vi "Write Data to HW.vi"(11 "Plugin in":refnum<class "Plugin.lvclass">) -> (0 "error out":errorcluster, 3 "Plugin out":refnum<class "Plugin.lvclass">)   [LabVIEW 2024, in "FPGA Addon Engine.lvlib" / "Plugin.lvclass"]
uses:
  Plugin.lvclass
  Plugin.lvclass/Plugin.ctl
  FPGA Addon Engine.lvlib
  VS Engine Abstraction/VS Engine Interface/VS Engine Interface.lvclass
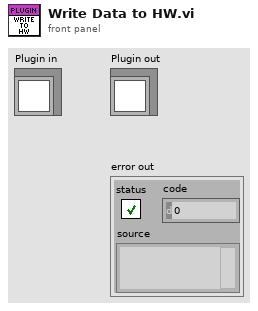
[diagram p1: front panel]
types:
  T1 = typedef "FPGA Addon Engine.lvlib/State Variables.ctl" = cluster{"FPGA Ref":refnum<k20>, "IncomingRegisters.Refs":T2[], "IncomingDMA.Refs":T5[], "OutgoingRegisters.Refs":T2[], "OutgoingDMA.Refs":T10[], "Compiled":T12}
  T2 = typedef "FPGA Addon Engine.lvlib/Register Settings.ctl" = cluster{"Name":string, "Data Type":T3, "session":u32, "Scalar Type":T4, "Index":i32, "Length":i32, "attributes":variant, "default value":variant, "RegisterOffset":u32}
  T3 = typedef "FPGA Addon Shared.lvlib/FPGA Addon Data Type.ctl" = enum8{"<Null>", "I8", "I16", "I32", "I64", "U8", "U16", "U32", "U64", "SGL", "Boolean", "Analog PWM In Settings", "Analog PWM In", "Digital PWM In Settings", "Digital PWM In", "Digital PWM Out", "Sine Out", "FXP", "FXP+/-24.5", "FXP+/-16.5", "FXP+/-32.8", "FXP+/-64.32", "FXP+/-16.7", "FXP+/-20.5", "FXP+/-27.5", "FXP+/-32.16", "FXP+16.3", "FXP+18.3", "Digital Static In", "Digital Static Out", "Digital Static In Settings", "Digital WSS Out", "Quad Encoder Settings", "Quad Encoder In", "Group"}
  T4 = typedef "FPGA Addon Shared.lvlib/Scalar Type.ctl" = enum16{"Standard", "Bitpacked"}
  T5 = typedef "FPGA Addon Engine.lvlib/DMA Input References.ctl" = cluster{"Addon Name":string, "Waveform Ref":refnum<class "Multiple Waveforms Write (DBL).lvclass">, "DMA Name":string, "DMA Settings":T6, "Refs":T9}
  T6 = typedef "FPGA Addon Shared.lvlib/DMA Settings.ctl" = cluster{"Number of Channels":u8, "Delacing Scheme":T7, "Update Rate":u32, "dt":dbl, "Mode":T8, "Number of Samples":u32, "DMA Host Buffer":u32}
  T7 = typedef "FPGA Addon Shared.lvlib/Delacing Scheme.ctl" = enum8{"Interleaved", "Bitpacked"}
  T8 = typedef "FPGA Addon Shared.lvlib/DMA Acquisition Mode.ctl" = enum8{"Continuous", "Triggered Finite"}
  T9 = typedef "FPGA Addon Engine.lvlib/DMA Input Refs.ctl" = cluster{"Data Type":T3, "DMA_SGL":refnum<k20>, "DMA_U64":refnum<k20>, "DMA_I64":refnum<k20>, "DMA_FXP+/-32.8":refnum<k20>, "DMA_FXP+/-64.32":refnum<k20>, "DMA_U32":refnum<k20>, "DMA_U16":refnum<k20>, "DMA_U8":refnum<k20>, "DMA_I32":refnum<k20>, "DMA_I16":refnum<k20>, "DMA_I8":refnum<k20>, "DMA_FXP+/-32.16":refnum<k20>}
  T10 = typedef "FPGA Addon Engine.lvlib/DMA Output References.ctl" = cluster{"Addon Name":string, "Waveforms":refnum<class "Single Waveform Read (DBL).lvclass">[], "DMA Name":string, "Refs":T11}
  T11 = typedef "FPGA Addon Engine.lvlib/DMA Output Refs.ctl" = cluster{"Data Type":T3, "DMA_SGL":refnum<k20>, "DMA_U64":refnum<k20>, "DMA_I64":refnum<k20>, "DMA_FXP+/-32.8":refnum<k20>, "DMA_FXP+/-64.32":refnum<k20>, "DMA_U32":refnum<k20>, "DMA_U16":refnum<k20>, "DMA_U8":refnum<k20>, "DMA_I32":refnum<k20>, "DMA_I16":refnum<k20>, "DMA_I8":refnum<k20>, "DMA_FXP+/-32.16":refnum<k20>}
  T12 = typedef "FPGA Addon Shared.lvlib/Compiled.Settings.ctl" = cluster{"Name":string, "IncomingRegisters.Settings":T13[], "IncomingRegisters.Refs":cluster{"Refs":T15[], "Values":dbl[]}, "OutgoingRegisters.Settings":T13[], "OutgoingRegisters.Refs":cluster{"Refs":T15[], "Values":dbl[]}, "Incoming.Size":i32, "Outgoing.Size":i32, "IncomingDMA.Settings":T17[], "OutgoingDMA.Settings":T17[], "FPGA.Settings":T19, "Target.Type":T20}
  T13 = typedef "FPGA Addon Shared.lvlib/Compiled.RegisterSettings.ctl" = cluster{"Scalar Type":T4, "Index":i32, "Length":i32, "Register":T14}
  T14 = typedef "FPGA Addon Shared.lvlib/Register Information.ctl" = cluster{"Name":string, "Data Type":T3, "Default Value":variant, "Attributes":variant}
  T15 = typedef "Custom Device API.lvlib/Block Data Reference.ctl" = cluster{"Data Reference":T16, "Offset":u64, "Length":u64}
  T16 = typedef "Custom Device API.lvlib/Data Reference.ctl" = i32
  T17 = typedef "FPGA Addon Shared.lvlib/Compiled.DMASettings.ctl" = cluster{"Name":string, "Data Type":T3, "DMA.Settings":T6, "DMA.VSRefs":T18[]}
  T18 = typedef "Custom Device API.lvlib/Waveform Data Reference.ctl" = i32
  T19 = typedef "FPGA Addon Shared.lvlib/FPGA Settings.ctl" = cluster{"Bitfile path":path, "RIO Device Address":string, "Group":bool}
  T20 = typedef "Custom Device API.lvlib/Custom Device Target Type.ctl" = enum16{"PharLap", "VxWorks", "Windows", "Linux_32_ARM", "Linux_x64"}
  T21 = cluster{"Vars":T1, "Async?":bool, "Async":refnum<class "VS Plugin Inline Async API.lvclass">}
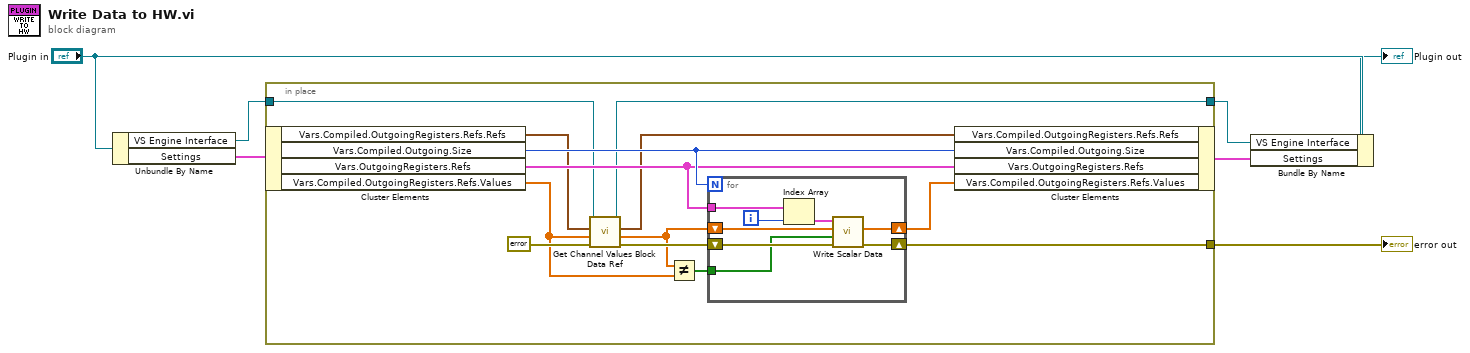
[diagram p0: block diagram]
diagram:
  n1 = Unbundle By Name("Plugin in") -> ("VS Engine Interface"=w2:refnum<class "VS Engine Interface.lvclass">, "Settings"=w7:T21)
  n2 = in-place {
    in-place-border: [w16] -> w3
    in-place-border: w2 -> [w13]
    in-place-border: [w8] -> w1
    n3 = in-place-cluster #1(w7) -> ("Vars.Compiled.OutgoingRegisters.Refs.Refs"=w12:T15[], "Vars.Compiled.Outgoing.Size"=w19:i32, "Vars.OutgoingRegisters.Refs"=w17:T2[], "Vars.Compiled.OutgoingRegisters.Refs.Values"=w11:dbl[])
    n4 = call-dynamic "Get Channel Values Block Data Ref.vi"("error in"=errorcluster {"status"=FALSE, "code"=0, "source"=""}, "Values Array in"=w11, "Block Data Ref"=w12, "VS Engine Interface in"=w13) -> ("error out"=w14:errorcluster, "Values Array out"=w9:dbl[], "Block Data Ref dup"=w10:T15[], "VS Engine Interface out"=w8:refnum<class "VS Engine Interface.lvclass">)  [unwired: 4 in]
    n5 = Not Equal?(x=w9, y=w11) -> (x != y?=w18:bool[])
    n6 = for {
      N: w19 -> [_]
      shift-right: [w22] -> w20
      shift-left: w9 -> [w27]
      shift-right: [w23] -> w16
      shift-left: w14 -> [w28]
      tunnel: w18 -> [w21]
      tunnel: w17 -> [w26]
      i -> [w24]
      n7 = Index Array(array=w26, index=w24) -> (element=w25:T2)
      n8 = call "Write Scalar Data.vi"("error in (no error)"=w28, "Changed?"=w21, "Values"=w27, "Cluster"=w25) -> ("error out"=w23:errorcluster, "Values"=w22:dbl[])  [unwired: 6 in]
    }
    n9 = in-place-cluster #1("Vars.Compiled.OutgoingRegisters.Refs.Refs"=w10, "Vars.Compiled.Outgoing.Size"=w19, "Vars.OutgoingRegisters.Refs"=w17, "Vars.Compiled.OutgoingRegisters.Refs.Values"=w20) -> (w5:T21)
  }
  "error out" <- w3
  n10 = Bundle By Name(cluster="Plugin in", "VS Engine Interface"=w1, "Settings"=w5) -> (→"Plugin out":refnum<class "Plugin.lvclass">)
